vi "AutoSimu (SubVI).vi"(8 "Deflection_Setting 5":dbl, 9 "Cycles_Setting":dbl, 10 "BEND. Moment_Setting":dbl, 11 "Tachometer_Setting":dbl) -> (0 "Deflection_Setting":dbl, 1 "Deflection_Setting 2":dbl, 2 "Deflection_Setting 3":dbl, 3 "Deflection_Setting 4":dbl)   [LabVIEW 2021]
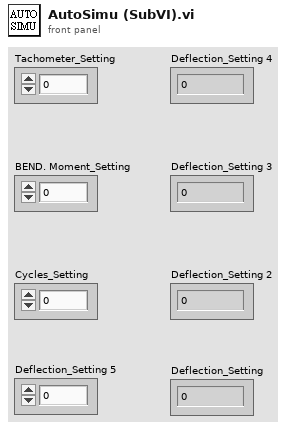
[diagram p1: front panel]
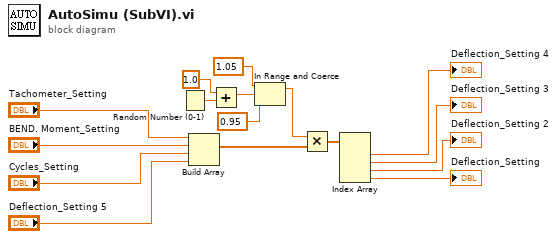
[diagram p0: block diagram]
diagram:
  n1 = Random Number (0-1)() -> (number: 0 to 1=w5:dbl)
  n2 = Build Array("Tachometer_Setting", "BEND. Moment_Setting", "Cycles_Setting", "Deflection_Setting 5") -> (w4:dbl[])
  n3 = Add(x=1.0, y=w5) -> (x+y=w14:dbl)
  n4 = In Range and Coerce(upper limit=1.05, x=w14, lower limit=0.95) -> (coerced(x)=w1:dbl)  [unwired: 1 out]
  n5 = Multiply(x=w1, y=w4) -> (x*y=w7:dbl[])
  n6 = Index Array(array=w7) -> (element #1=→"Deflection_Setting 4":dbl, element #2=→"Deflection_Setting 3":dbl, element #3=→"Deflection_Setting 2":dbl, element #4=→"Deflection_Setting":dbl)  [unwired: 4 in]
